vi "GaussianKernel7x7.vi"() -> (2 "appended array":dbl[][](array[numeric]))   [LabVIEW 2022 SP3]
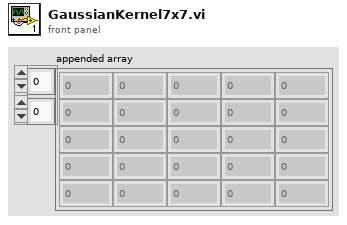
[diagram p1: front panel]
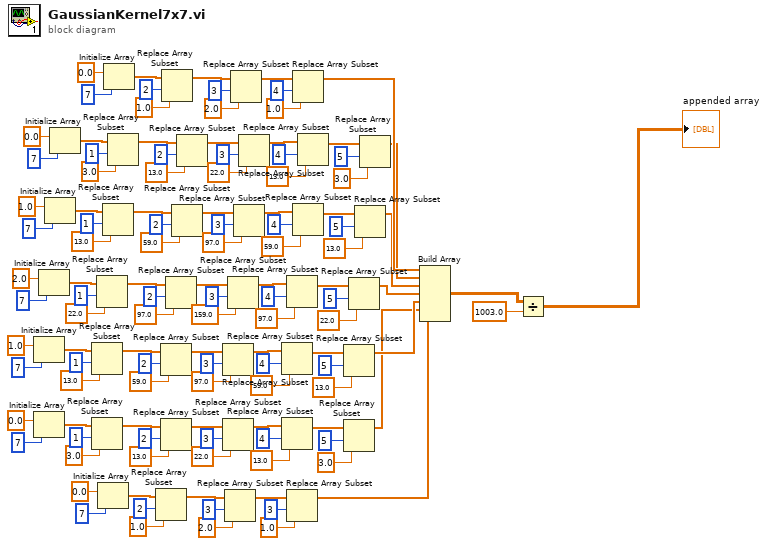
[diagram p0: block diagram]
diagram:
  n1 = Initialize Array(1.0 ("element"), 7 ("dimension size")) -> (w37:dbl[])
  n2 = Initialize Array(0.0 ("element"), 7 ("dimension size")) -> (w20:dbl[])
  n3 = Initialize Array(2.0 ("element"), 7 ("dimension size")) -> (w54:dbl[])
  n4 = Initialize Array(1.0 ("element"), 7 ("dimension size")) -> (w71:dbl[])
  n5 = Initialize Array(0.0 ("element"), 7 ("dimension size")) -> (w88:dbl[])
  n6 = Replace Array Subset(array=w37, new element=13.0 ("new element/subarray"), index=1) -> (w36:dbl[])
  n7 = Replace Array Subset(array=w20, new element=3.0 ("new element/subarray"), index=1) -> (w19:dbl[])
  n8 = Replace Array Subset(array=w54, new element=22.0 ("new element/subarray"), index=1) -> (w53:dbl[])
  n9 = Initialize Array(0.0 ("element"), 7 ("dimension size")) -> (w99:dbl[])
  n10 = Replace Array Subset(array=w71, new element=13.0 ("new element/subarray"), index=1) -> (w70:dbl[])
  n11 = Initialize Array(0.0 ("element"), 7 ("dimension size")) -> (w113:dbl[])
  n12 = Replace Array Subset(array=w88, new element=3.0 ("new element/subarray"), index=1) -> (w87:dbl[])
  n13 = Replace Array Subset(array=w99, new element=1.0 ("new element/subarray"), index=2) -> (w98:dbl[])
  n14 = Replace Array Subset(array=w36, new element=59.0 ("new element/subarray"), index=2) -> (w33:dbl[])
  n15 = Replace Array Subset(array=w19, new element=13.0 ("new element/subarray"), index=2) -> (w16:dbl[])
  n16 = Replace Array Subset(array=w113, new element=1.0 ("new element/subarray"), index=2) -> (w112:dbl[])
  n17 = Replace Array Subset(array=w53, new element=97.0 ("new element/subarray"), index=2) -> (w50:dbl[])
  n18 = Replace Array Subset(array=w70, new element=59.0 ("new element/subarray"), index=2) -> (w67:dbl[])
  n19 = Replace Array Subset(array=w87, new element=13.0 ("new element/subarray"), index=2) -> (w84:dbl[])
  n20 = Replace Array Subset(array=w33, new element=97.0 ("new element/subarray"), index=3) -> (w30:dbl[])
  n21 = Replace Array Subset(array=w16, new element=22.0 ("new element/subarray"), index=3) -> (w13:dbl[])
  n22 = Replace Array Subset(array=w98, new element=2.0 ("new element/subarray"), index=3) -> (w95:dbl[])
  n23 = Replace Array Subset(array=w50, new element=159.0 ("new element/subarray"), index=3) -> (w47:dbl[])
  n24 = Replace Array Subset(array=w112, new element=2.0 ("new element/subarray"), index=3) -> (w109:dbl[])
  n25 = Replace Array Subset(array=w67, new element=97.0 ("new element/subarray"), index=3) -> (w64:dbl[])
  n26 = Replace Array Subset(array=w84, new element=22.0 ("new element/subarray"), index=3) -> (w81:dbl[])
  n27 = Replace Array Subset(array=w30, new element=59.0 ("new element/subarray"), index=4) -> (w25:dbl[])
  n28 = Replace Array Subset(array=w13, new element=13.0 ("new element/subarray"), index=4) -> (w8:dbl[])
  n29 = Replace Array Subset(array=w47, new element=97.0 ("new element/subarray"), index=4) -> (w42:dbl[])
  n30 = Replace Array Subset(array=w95, new element=1.0 ("new element/subarray"), index=3) -> (w1:dbl[])
  n31 = Replace Array Subset(array=w109, new element=1.0 ("new element/subarray"), index=4) -> (w7:dbl[])
  n32 = Replace Array Subset(array=w64, new element=59.0 ("new element/subarray"), index=4) -> (w59:dbl[])
  n33 = Replace Array Subset(array=w81, new element=13.0 ("new element/subarray"), index=4) -> (w76:dbl[])
  n34 = Replace Array Subset(array=w25, new element=13.0 ("new element/subarray"), index=5) -> (w3:dbl[])
  n35 = Replace Array Subset(array=w8, new element=3.0 ("new element/subarray"), index=5) -> (w2:dbl[])
  n36 = Replace Array Subset(array=w42, new element=22.0 ("new element/subarray"), index=5) -> (w4:dbl[])
  n37 = Replace Array Subset(array=w59, new element=13.0 ("new element/subarray"), index=5) -> (w5:dbl[])
  n38 = Replace Array Subset(array=w76, new element=3.0 ("new element/subarray"), index=5) -> (w6:dbl[])
  n39 = Build Array(w7, w6, w5, w4, w3, w2, w1) -> (w105:dbl[][])
  n40 = Divide(x=w105, y=1003.0) -> (x/y=→"appended array":dbl[][])
